vi "time2name.vi"(1 "timestamp":timestamp, 3 "DevNo":i32, 4 "ext":string="tdms") -> (0 "String":string)   [LabVIEW 2010]
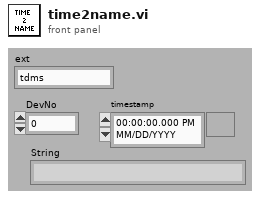
[diagram p1: front panel]
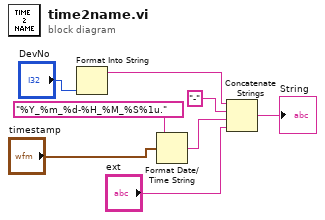
[diagram p0: block diagram]
diagram:
  n1 = Format Into String("DevNo") -> (resulting string=w7:string)  [unwired: 3 in, 1 out]
  n2 = Format Date/Time String(time format string (%c)="%Y_%m_%d-%H_%M_%S%1u.", seconds (now)="timestamp") -> (date/time string=w8:string)  [unwired: 1 in]
  n3 = Concatenate Strings(w7, "-" ("string"), w8, "ext") -> (→"String":string)
